vi "WriteHardwareInfoUSB.vi"(8 "error in (no error)":errorcluster, 11 "path":path) -> (0 "error out":errorcluster)   [LabVIEW 2017, in "USBDrive.lvlib"]
uses:
  <vilib>/addons/InsightCM/Devices/Shared/Common/USBDrive/USBDrive.lvlib
  <vilib>/addons/SystemInfoProcess/SystemInfoProcess.lvlib
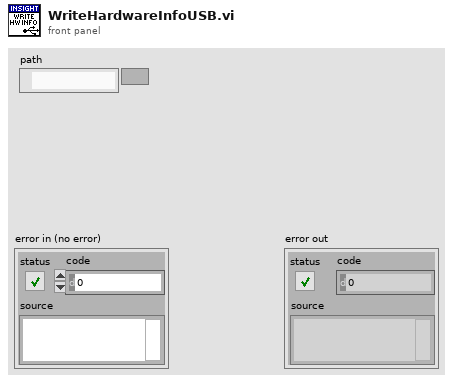
[diagram p1: front panel]
types:
  T1 = typedef "cRIODetectHW.lvlib/SystemHW.ctl" = cluster{"controller":T2, "chassis":T2, "modules":T2[]}
  T2 = typedef "cRIODetectHW.lvlib/cRIO Product Info.ctl" = cluster{"vendorName":string, "productName":string, "serialNumber":string}
  T3 = typedef "KeyValuePair.ctl" = cluster{"Key":string, "Value":string}
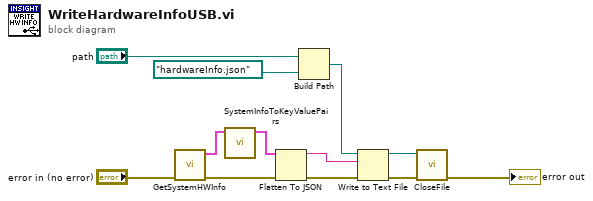
[diagram p0: block diagram]
diagram:
  n1 = call <vilib>:"GetSystemHWInfo.vi"("error in (no error)"="error in (no error)") -> ("error out"=w8:errorcluster, "system info"=w10:T1)  [unwired: 8 in, 1 out]
  n2 = call "SystemInfoToKeyValuePairs.vi"("system info"=w10) -> ("hardware info key value pair"=w11:T3[])  [unwired: 10 in]
  n3 = Flatten To JSON(anything=w11, error in (no error)=w8) -> (JSON string=w7:string, 11:w9:errorcluster)  [unwired: 1 in]
  n4 = Build Path(base path="path", name or relative path=path "hardwareInfo.json" ("dup path")) -> (appended path=w12:path)
  n5 = Write to Text File(file (use dialog)=w12, text=w7, error in=w9) -> (refnum out=w3:refnum<file>, error out=w2:errorcluster)  [unwired: 1 in, 1 out]
  n6 = call <vilib>:"CloseFile.vi"("error in (no error)"=w2, "file reference"=w3) -> ("error out"=→"error out":errorcluster)  [unwired: 9 in]
